vi "groundtruth_position.vi"(11 "Refnum in":refnum<k20>) -> (2 "state":cluster{"X":sgl, "Y":sgl, "Theta":dbl})   [LabVIEW 2016]
uses:
  <resource>/objmgr/LVODE.rc
  <vilib>/robotics/Kinematics/NI_Kinematics.lvlib
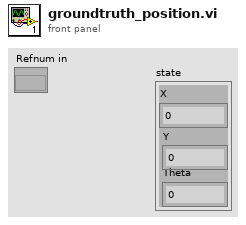
[diagram p1: front panel]
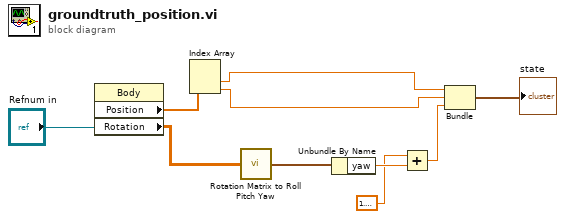
[diagram p0: block diagram]
diagram:
  n1 = property class="Body"(reference="Refnum in") -> ("Position"=w9:sgl[], "Rotation"=w6:sgl[][])  [unwired: 1 in, 2 out]
  n2 = Index Array(array=w9) -> (element #1=w8:sgl, element #2=w7:sgl)  [unwired: 2 in]
  n3 = call <vilib>:"Rotation Matrix to Roll Pitch Yaw.vi"("rotation matrix"=w6) -> ("angles"=w5:cluster{"roll":dbl, "pitch":dbl, "yaw":dbl})
  n4 = Unbundle By Name(w5) -> ("yaw"=w4:dbl)
  n5 = Add(x=1.5707963267948966, y=w4) -> (x+y=w2:dbl)
  n6 = Bundle(w8, w7, w2) -> (→"state":cluster{sgl, sgl, dbl})  [unwired: 1 in]
